vi "sCMOS_init_ramp.vi"(3 "error in":errorcluster, 4 "data cluster":T1, 5 "handle":u32) -> (0 "error out":errorcluster {"code" format="%.0x"}, 2 "Ready?":bool)   [LabVIEW 2015]
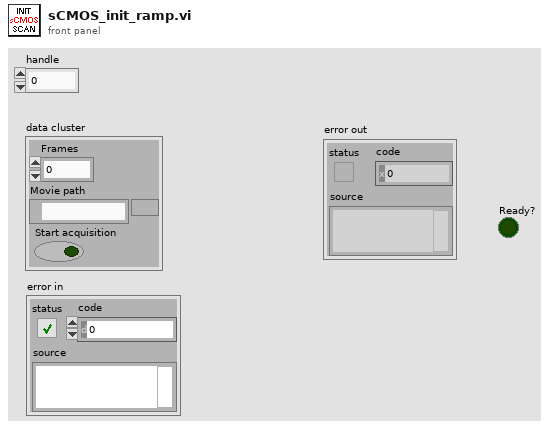
[diagram p1: front panel]
types:
  T1 = cluster{"Frames":i32, "Movie path":path, "Start acquisition":bool}
  T2 = cluster{"Mode":u32, "Polarity":u32, "Times":u32, "Delay":dbl}
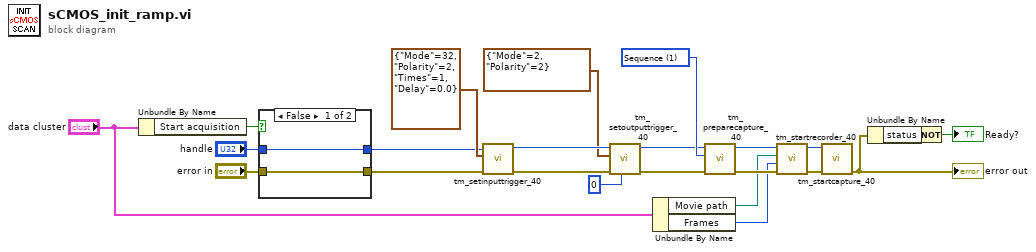
[diagram p0: block diagram]
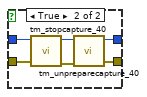
[diagram p2: hidden frame]
diagram:
  w19 = 1 items=["Snap", "Sequence"] ("Capture mode")
  n1 = Unbundle By Name("data cluster") -> ("Start acquisition"=w15:bool)
  n2 = case shown="False" w15 {
    tunnel: "error in" -> [w25 w31]
    tunnel: [w25 w27] -> w1
    tunnel: "handle" -> [w24 w30]
    tunnel: [w24 w26] -> w2
    frame False {
    }
    frame True {
      n3 = call <userlib>:"tm_stopcapture_40.vi"("error in (no error)"=w31, "Handle in"=w30) -> ("error out"=w29:errorcluster, "Handle out"=w28:u32)  [unwired: 8 in]
      n4 = call <userlib>:"tm_unpreparecapture_40.vi"("error in (no error)"=w29, "Handle in"=w28) -> ("error out"=w27:errorcluster, "Handle out"=w26:u32)  [unwired: 8 in]
    }
  }
  n5 = call <userlib>:"tm_setinputtrigger_40.vi"("error in (no error)"=w1, "Parameters"=T2 {"Mode"=32, "Polarity"=2, "Times"=1, "Delay"=0.0}, "Handle in"=w2) -> ("error out"=w13:errorcluster, "Handle out"=w11:u32)  [unwired: 7 in]
  n6 = call <userlib>:"tm_setoutputtrigger_40.vi"("Port"=0, "error in (no error)"=w13, "Type"=cluster{"Mode":u32, "Polarity":u32} {"Mode"=2, "Polarity"=2}, "Handle in"=w11) -> ("error out"=w12:errorcluster, "Handle out"=w10:u32)  [unwired: 6 in]
  n7 = Unbundle By Name("data cluster") -> ("Movie path"=w7:path, "Frames"=w14:i32)
  n8 = call <userlib>:"tm_preparecapture_40.vi"("error in (no error)"=w12, "Capture mode"=w19, "Handle in"=w10) -> ("error out"=w20:errorcluster, "Handle out"=w21:u32)  [unwired: 5 in, 2 out]
  n9 = call <userlib>:"tm_startrecorder_40.vi"("error in (no error)"=w20, "frames"=w14, "File"=w7, "Handle in"=w21) -> ("error out"=w22:errorcluster, "Handle out"=w23:u32)  [unwired: 6 in]
  n10 = call <userlib>:"tm_startcapture_40.vi"("error in (no error)"=w22, "Handle in"=w23) -> ("error out"=w6:errorcluster)  [unwired: 8 in, 1 out]
  "error out" <- w6
  n11 = Unbundle By Name(w6) -> ("status"=w5:bool)
  n12 = Not(x=w5) -> (.not. x?=→"Ready?":bool)
